vi "disconnect.vi"(0 "DB Session ID":i32, 11 "error in (no error)":errorcluster) -> (15 "error out":errorcluster)   [LabVIEW 2017, in "Database.lvlib"]
uses:
  Database.lvlib
  bin/Database.dll
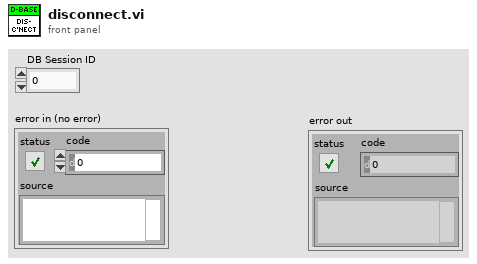
[diagram p1: front panel]
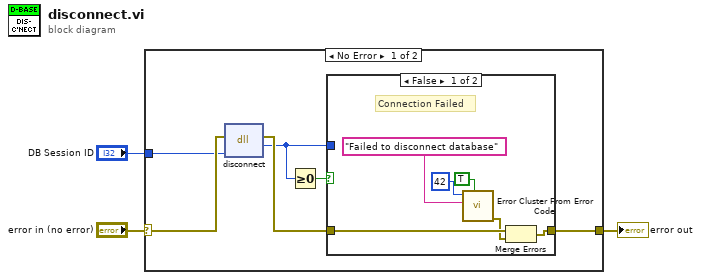
[diagram p0: block diagram]
diagram:
  n1 = case shown="No Error" "error in (no error)" {
    selector: "error in (no error)" -> [w9 w17]
    tunnel: [w5 w17] -> w2
    tunnel: "DB Session ID" -> [w4 _]
    frame No Error {
      n2 = dll-call lib="C:/Users/Caleb/Desktop/nebraska-silicon-lab/pixel-gantry-extra/LV/bin/Database.dll" fn="disconnect"(error in=w9, "conn_id"=w4) -> (error out=w7:errorcluster, "return type"=w6:i32)  [unwired: 3 in, 1 out]
      n3 = Greater Or Equal To 0?(x=w6) -> (x >= 0?=w8:bool)
      n4 = case shown="False" w8 {
        tunnel: w7 -> [w15 w16]
        tunnel: w6 -> [_ _]
        tunnel: [w14 w16] -> w5
        frame False {
          # "Connection Failed"
          n5 = call <vilib>:"Error Cluster From Error Code.vi"("show call chain? (False)"=TRUE, "error message (\"\")"="Failed to disconnect database" ("error message (\"\")"), "error code (0)"=42) -> ("error out"=w13:errorcluster)  [unwired: 6 in]
          n6 = Merge Errors(w15, w13) -> (w14:errorcluster)
        }
        frame True {
          # "Connection Successful"
        }
      }
    }
    frame Error {
    }
  }
  "error out" <- w2
